vi "moving_object.vi"() -> ()   [LabVIEW 2023]
uses:
  <vilib>/Utility/miscctls.llb/LVRectTypeDef.ctl
  <vilib>/Utility/miscctls.llb/LVPositionTypeDef.ctl
panel:
  out "current pos":cluster{"Left":i32, "Top":i32}
  out "final pos":cluster{"Left":i32, "Top":i32}
  out "initial pos":cluster{"Left":i32, "Top":i32}
  out "step size":i32
  out "Camera":bool
  in  "Stop":bool
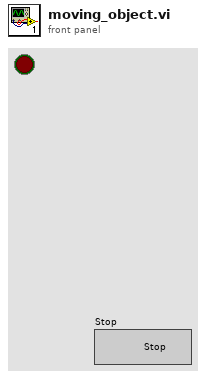
[diagram p1: front panel]
types:
  T1 = typedef "LVPositionTypeDef.ctl" = cluster{"Left":i32, "Top":i32}
  T2 = typedef "LVRectTypeDef.ctl" = cluster{"Left":i16, "Top":i16, "Right":i16, "Bottom":i16}
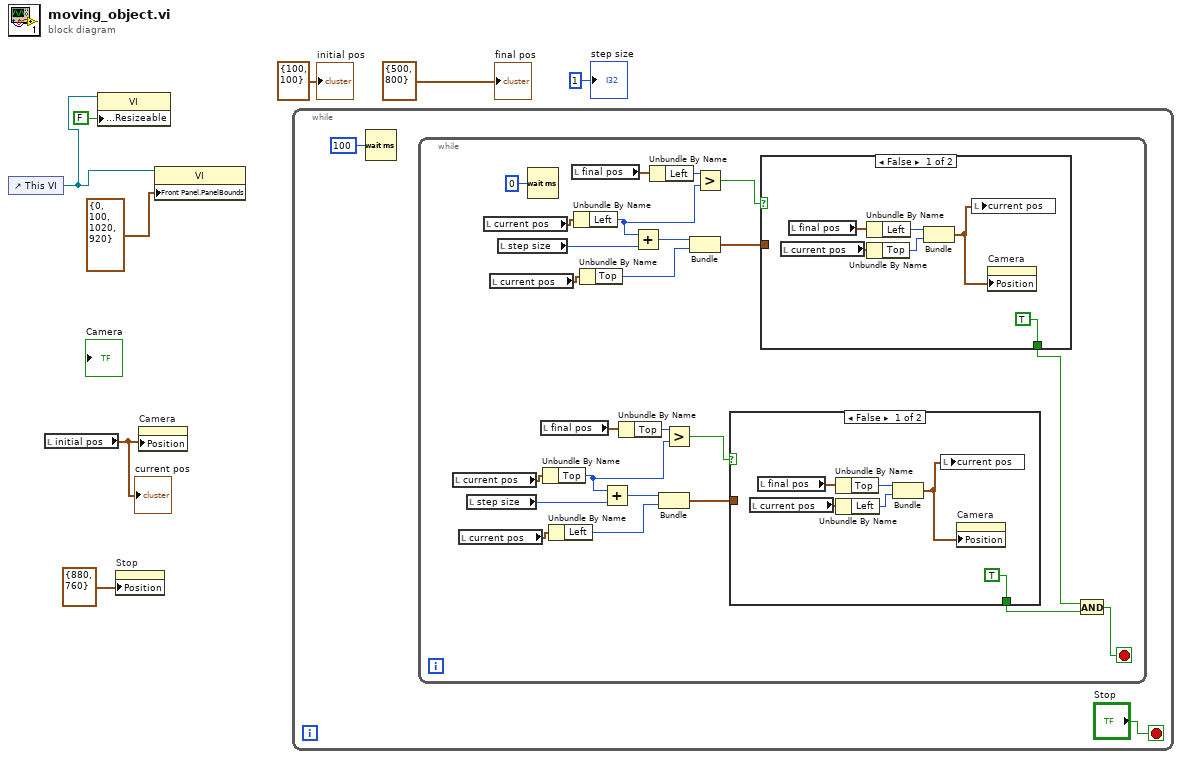
[diagram p0: block diagram]
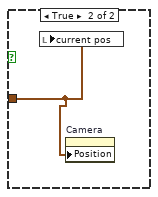
[diagram p2: hidden frame]
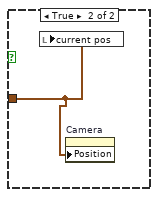
[diagram p3: hidden frame]
diagram:
  n1 = control-ref of="This VI"() -> (w5:refnum<vi>)
  n2 = local read "initial pos"() -> (w2:cluster{"Left":i32, "Top":i32})
  "current pos" <- w2
  n3 = property class="VI"(reference=w5, "Front Panel.Resizeable"=FALSE ("Front Panel Window:Resizable")) -> ()  [unwired: 1 in, 2 out]
  n4 = property on="Stop" class="Bool"("Position"=T1 {"Left"=880, "Top"=760}) -> ()  [unwired: 2 in, 2 out]
  n5 = property on="Camera" class="Bool (strict)"("Position"=w2) -> ()  [unwired: 2 in, 2 out]
  n6 = property class="VI"(reference=w5, "Front Panel.PanelBounds"=T2 {"Left"=0, "Top"=100, "Right"=1020, "Bottom"=920} ("Front Panel Window:Panel Bounds")) -> ()  [unwired: 1 in, 2 out]
  n7 = while {
    stop <- "Stop" stop-if-true
    n8 = Wait (ms)(milliseconds to wait=u32 100) -> ()  [unwired: 1 out]
    n9 = while {
      stop <- w11 stop-if-true
      n10 = local read "current pos"() -> (w23:cluster{"Left":i32, "Top":i32})
      n11 = local read "current pos"() -> (w21:cluster{"Left":i32, "Top":i32})
      n12 = local read "step size"() -> (w22:i32)
      n13 = local read "current pos"() -> (w34:cluster{"Left":i32, "Top":i32})
      n14 = local read "current pos"() -> (w32:cluster{"Left":i32, "Top":i32})
      n15 = local read "step size"() -> (w33:i32)
      n16 = Wait (ms)(milliseconds to wait=u32 0) -> ()  [unwired: 1 out]
      n17 = local read "final pos"() -> (w17:cluster{"Left":i32, "Top":i32})
      n18 = Unbundle By Name(w23) -> ("Top"=w15:i32)
      n19 = Unbundle By Name(w21) -> ("Left"=w19:i32)
      n20 = local read "final pos"() -> (w27:cluster{"Left":i32, "Top":i32})
      n21 = Unbundle By Name(w34) -> ("Left"=w25:i32)
      n22 = Unbundle By Name(w32) -> ("Top"=w30:i32)
      n23 = Add(x=w15, y=w22) -> (x+y=w20:i32)
      n24 = Unbundle By Name(w17) -> ("Top"=w16:i32)
      n25 = Add(x=w25, y=w33) -> (x+y=w31:i32)
      n26 = Unbundle By Name(w27) -> ("Left"=w26:i32)
      n27 = Bundle(w20, "Left"=w19) -> (w18:cluster{i32, "Left":i32})  [unwired: 1 in]
      n28 = Greater?(x=w16, y=w15) -> (0:w14:bool)
      n29 = Bundle(w31, "Top"=w30) -> (w29:cluster{i32, "Top":i32})  [unwired: 1 in]
      n30 = Greater?(x=w26, y=w25) -> (0:w24:bool)
      n31 = case shown="False" w14 {
        tunnel: w18 -> [_ w41]
        tunnel: [TRUE _] -> w12
        frame False {
          n32 = local read "current pos"() -> (w39:cluster{"Left":i32, "Top":i32})
          n33 = local read "final pos"() -> (w40:cluster{"Left":i32, "Top":i32})
          n34 = Unbundle By Name(w40) -> ("Top"=w38:i32)
          n35 = Unbundle By Name(w39) -> ("Left"=w37:i32)
          n36 = Bundle("Top"=w38, "Left"=w37) -> (w36:cluster{"Top":i32, "Left":i32})  [unwired: 1 in]
          n37 = local write "current pos"(w36) -> ()
          n38 = property on="Camera" class="Bool (strict)"("Position"=w36) -> ()  [unwired: 2 in, 2 out]
        }
        frame True {
          n39 = local write "current pos"(w41) -> ()
          n40 = property on="Camera" class="Bool (strict)"("Position"=w41) -> ()  [unwired: 2 in, 2 out]
        }
      }
      n41 = case shown="False" w24 {
        tunnel: w29 -> [_ w48]
        tunnel: [TRUE _] -> w13
        frame False {
          n42 = local read "current pos"() -> (w46:cluster{"Left":i32, "Top":i32})
          n43 = local read "final pos"() -> (w47:cluster{"Left":i32, "Top":i32})
          n44 = Unbundle By Name(w47) -> ("Left"=w45:i32)
          n45 = Unbundle By Name(w46) -> ("Top"=w44:i32)
          n46 = Bundle("Left"=w45, "Top"=w44) -> (w43:cluster{"Left":i32, "Top":i32})  [unwired: 1 in]
          n47 = local write "current pos"(w43) -> ()
          n48 = property on="Camera" class="Bool (strict)"("Position"=w43) -> ()  [unwired: 2 in, 2 out]
        }
        frame True {
          n49 = local write "current pos"(w48) -> ()
          n50 = property on="Camera" class="Bool (strict)"("Position"=w48) -> ()  [unwired: 2 in, 2 out]
        }
      }
      n51 = And(x=w13, y=w12) -> (x .and. y?=w11:bool)
    }
  }
  "step size" <- 1 ("step size")
  "initial pos" <- cluster{"Left":i32, "Top":i32} {"Left"=100, "Top"=100} ("initial pos")
  "final pos" <- cluster{"Left":i32, "Top":i32} {"Left"=500, "Top"=800} ("final pos")
